vi "cs-scanning-dirty.vi"() -> ()   [LabVIEW 2017]
uses:
  raster-scan-params.ctl
  controls/PI-params.ctl
  controls/boolean_info.ctl
  <vilib>/rvi/Emulation/niFpgaGetClockAttributes.vi
  <vilib>/rvi/Emulation/niFpgaSctlEmulationGetInTimedLoop.vi
  <vilib>/rvi/Emulation/niFpgaEmulationReportErrorSimple.vi
  <vilib>/rvi/Emulation/niFpgaProcessEmulError.vi
  <vilib>/rvi/eio/common/nirviEmuTemplateMethod_errors.vi
  <vilib>/rvi/Emulation/niFpgaEmulationIsFPGAContextNoSignature.vi
  <vilib>/rvi/DataTransferAndStorage/Container/Common/niFpgaContainerGetUniqueNameForEmu.vi
  <vilib>/rvi/Memory/Memory_Emulation/niFpgaMemoryEmulationCacheClearOnFirstRun.vi
  <vilib>/rvi/Memory/Memory_Emulation/nirvimemoryEmulationManagerCache_MakeExclusive.vi
  <vilib>/rvi/Memory/Memory_Emulation/niFpgaMemoryEmulationValidateCache.vi
  <vilib>/rvi/Memory/Memory_Emulation/nirvimemoryEmulationManagerCache_InsertValue.vi
  <vilib>/Utility/error.llb/Clear Errors.vi
  <vilib>/rvi/Memory/Memory_Emulation/nirvimemoryEmulationManagerCache_ReleaseExclusive.vi
  <vilib>/rvi/Memory/Memory_Emulation/nirvimemoryEmulationManagerCache_GetValue.vi
  <vilib>/rvi/Memory/Memory_Emulation/nirvimemoryEmulationManagerCache_SetValue.vi
  <vilib>/rvi/DataTransferAndStorage/Container/Common/niFpgaContainerExecOnDevCompGetState.vi
  <vilib>/rvi/Emulation/niFpgaCriticalErrorInLSC.vi
  <vilib>/eio/EIONode/EIONode.xnode
  <vilib>/rvi/DataTransferAndStorage/Container/XNode/niFpgaContainer.xnode
  <vilib>/rvi/DataTransferAndStorage/Register/Emulation/niFpgaRegisterEmulation.vi
  <vilib>/rvi/DataTransferAndStorage/Register/Emulation/niFpgaRegisterEmulationRefIn.vi
  libimaging-cs.lvlib
  FPGA-data-logging.lvlib
panel:
  out "number-settled-samples-Z":i16
  in  "Z-error-threshold":sgl format="%#_13g"
  in  "Z-settled-samples\nthreshold":i16
  out "number-settled-samples-y":i16
  out "number-settled-samples-x":i16
  in  "error-threshold":sgl format="%#_13g"
  in  "settled-samples\nthreshold":i16
  out "case-selected":i16
  out "z-DAC":sgl
  in  "numEntities":i16
  in  "ABORT":bool
  in  "Ki-xy":sgl=0.001 format="%#_13g"
  in  "z-bound":sgl
  in  "xy-bound":sgl
  out "boolean indicators":T1
  out "loggin-fifo-TO":bool=TRUE
  out "input-fifo-TO":bool=TRUE
  in  "raster-scan-params":T2={"TsTicks"=1600, "Stop"=TRUE, "TOL"=0.3, "ramp-rate"=0.0, "z-u-max"=5.0, "PI-params"={"Ki"=0.001, "setpoint"=0.0}} {"z-u-max" format="%#_13g"; "TOL" format="%#_13g"}
  in  "init Z up":fxp<+/-,16,5>
  in  "u_z(0)":sgl
  out "ADC-zaxis":fxp<+/-,24,5>
  out "e(0) (threshhold init)":fxp<+/-,16,5>
  out "xref ?":sgl=0.001 format="%#_13g"
  in  "z_UP":fxp<+/-,16,5>
  in  "zup-N":i16
  out "yref ?":sgl=0.001 format="%#_13g"
  in  "trigger-0":bool
  in  "initial case":i16=2
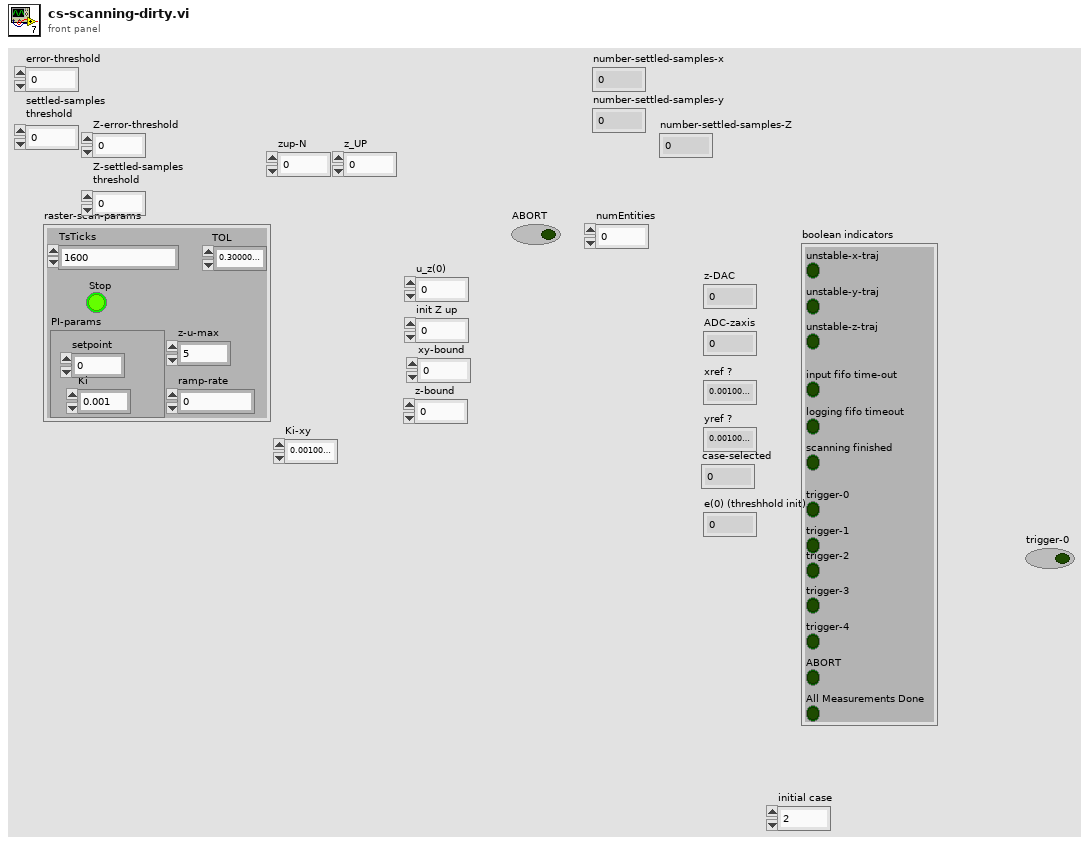
[diagram p1: front panel]
types:
  T1 = typedef "boolean_info.ctl" = cluster{"unstable-z-traj":bool, "input fifo time-out":bool, "logging fifo timeout":bool, "scanning finished":bool, "trigger-1":bool, "trigger-0":bool, "trigger-2":bool, "trigger-3":bool, "trigger-4":bool, "unstable-x-traj":bool, "unstable-y-traj":bool, "ABORT":bool, "All Measurements Done":bool}
  T2 = typedef "raster-scan-params.ctl" = cluster{"TsTicks":u32, "Stop":bool, "TOL":sgl, "ramp-rate":sgl, "z-u-max":sgl, "PI-params":T3}
  T3 = typedef "PI-params.ctl" = cluster{"Ki":sgl, "setpoint":sgl}
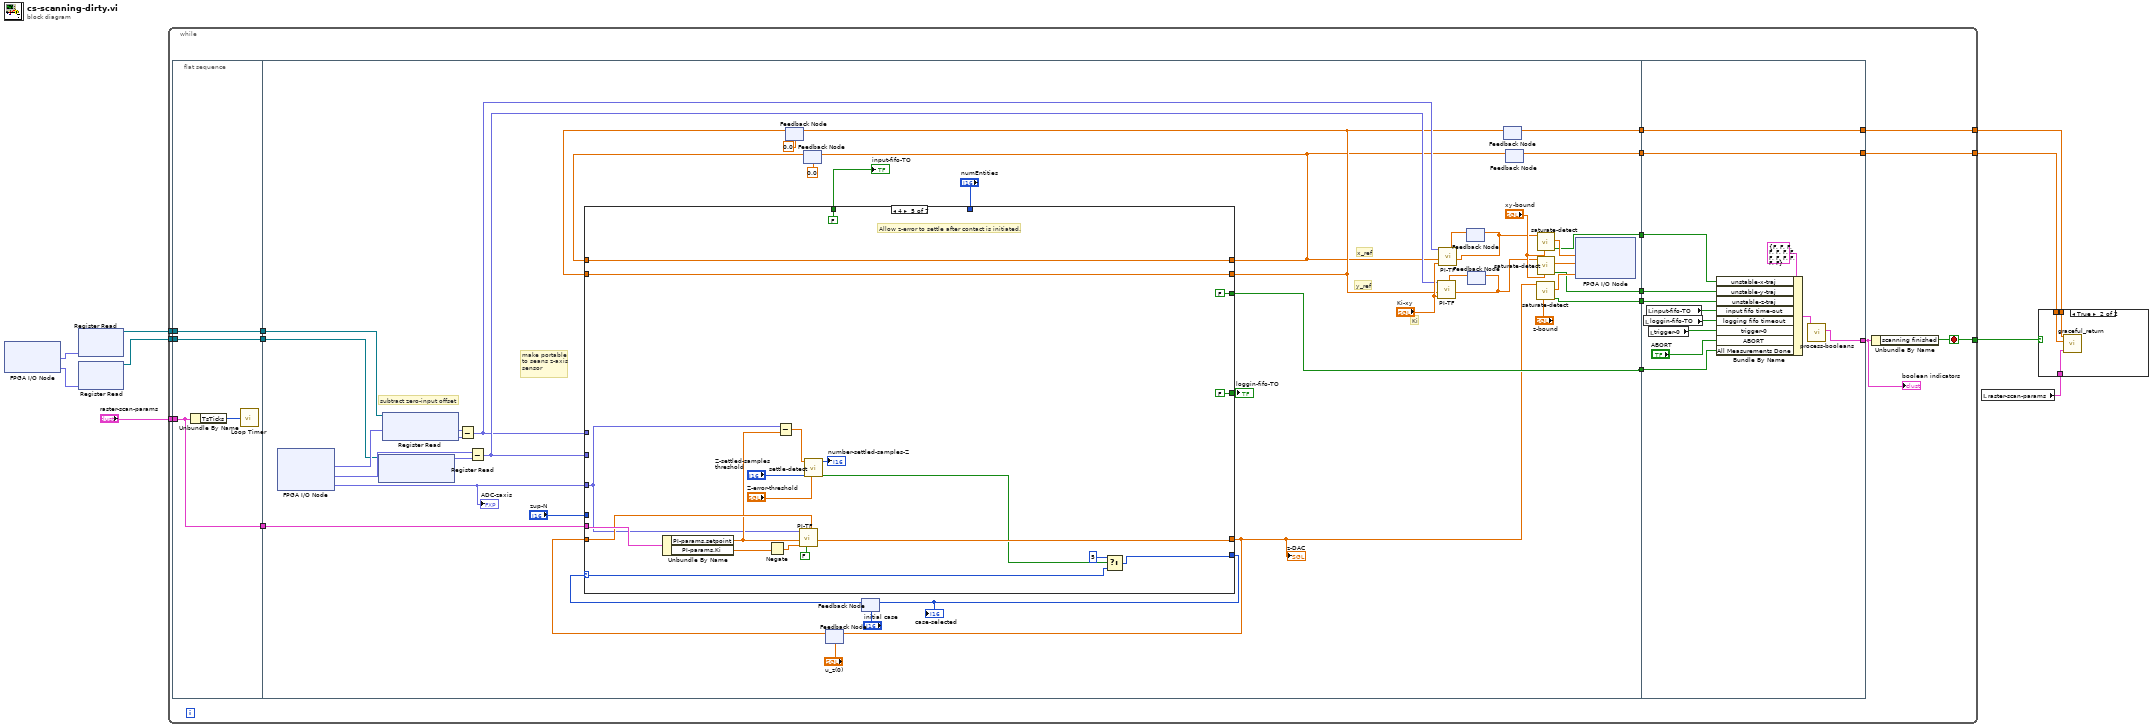
[diagram p0: block diagram]
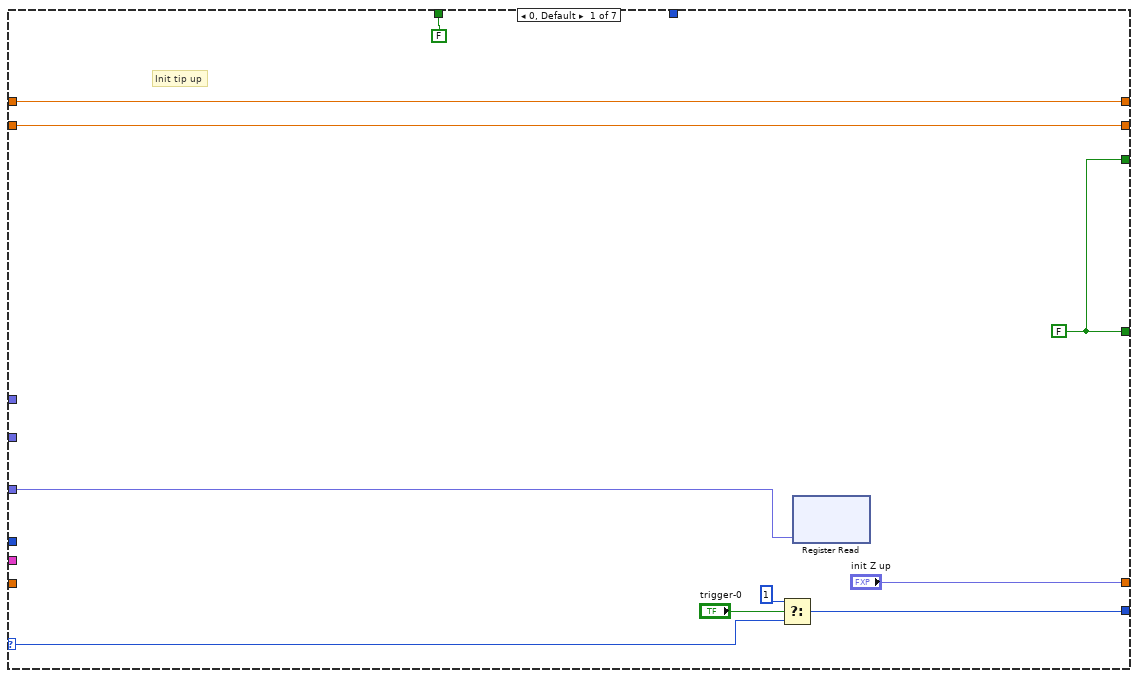
[diagram p3: hidden frame]
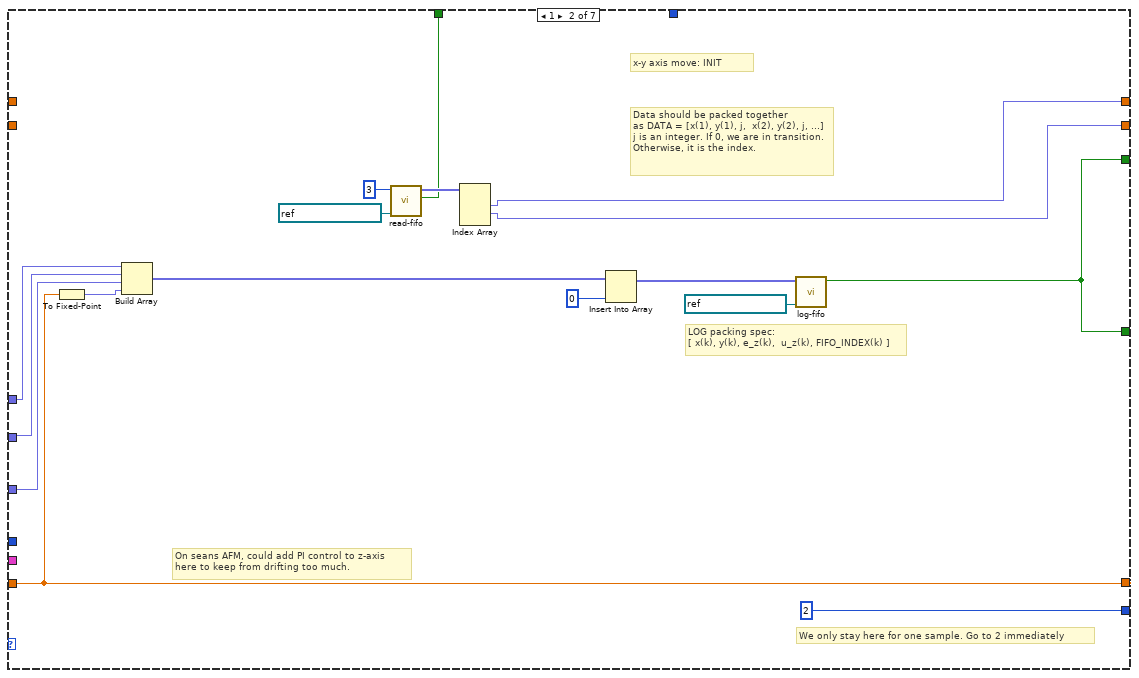
[diagram p4: hidden frame]
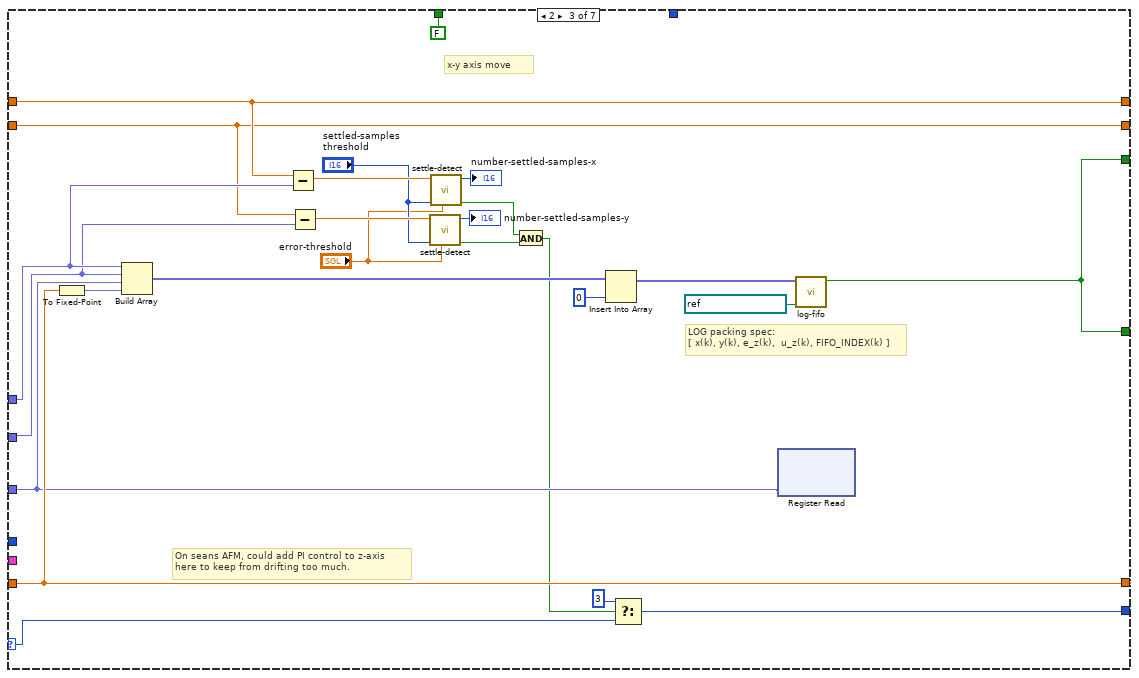
[diagram p5: hidden frame]
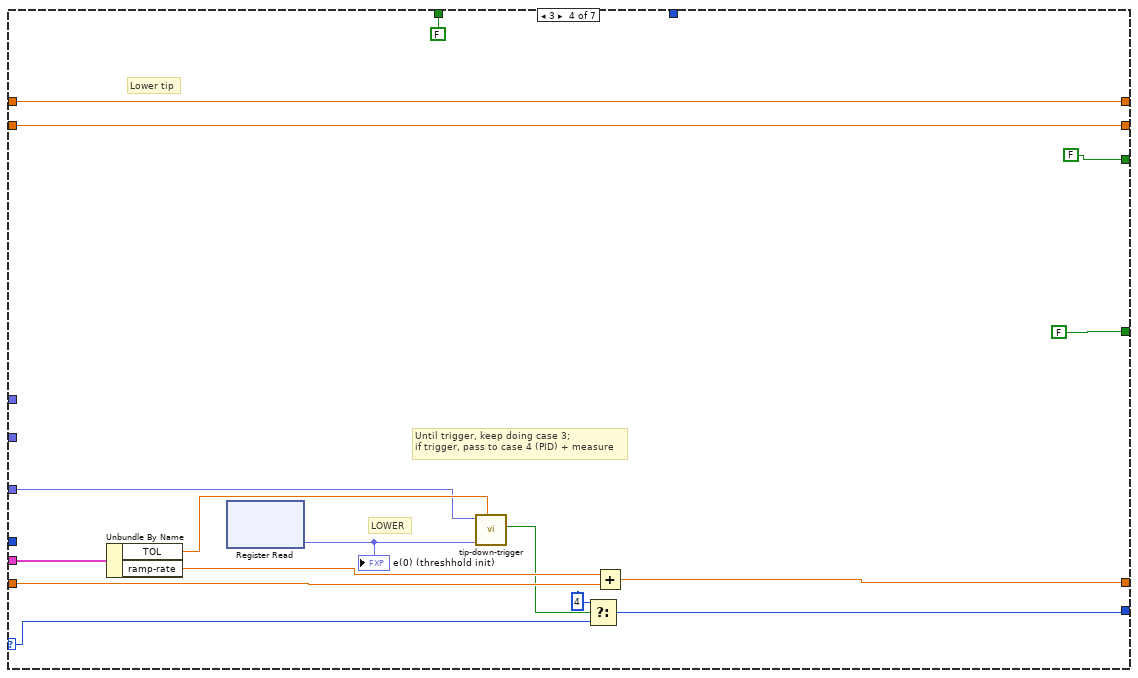
[diagram p6: hidden frame]
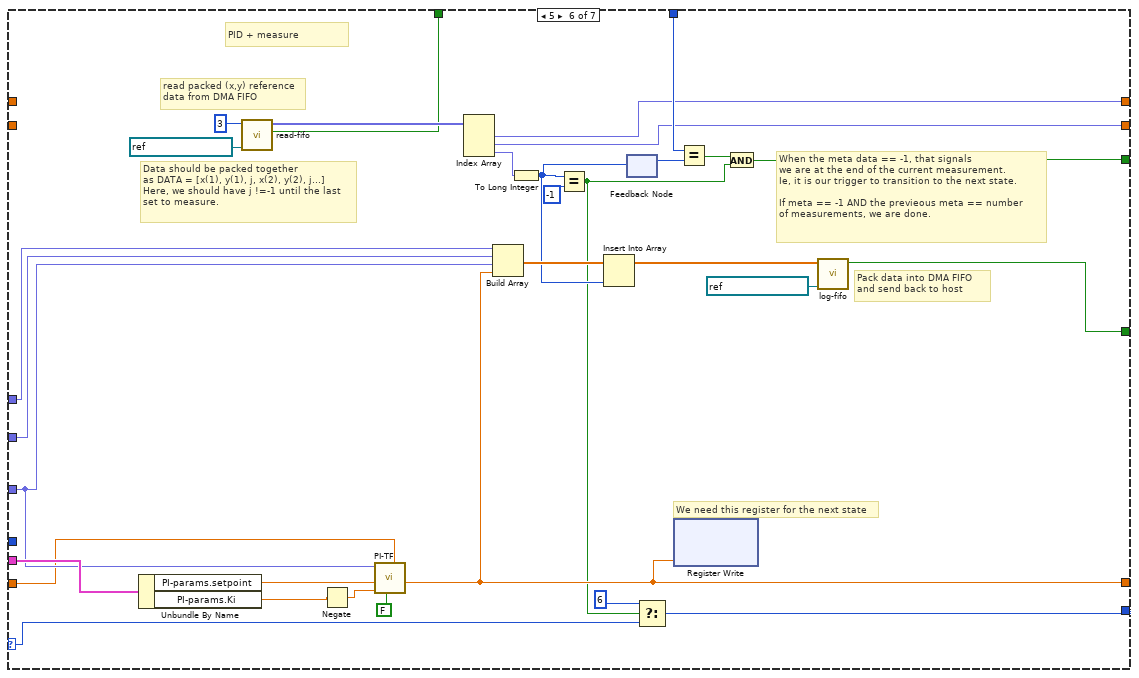
[diagram p7: hidden frame]
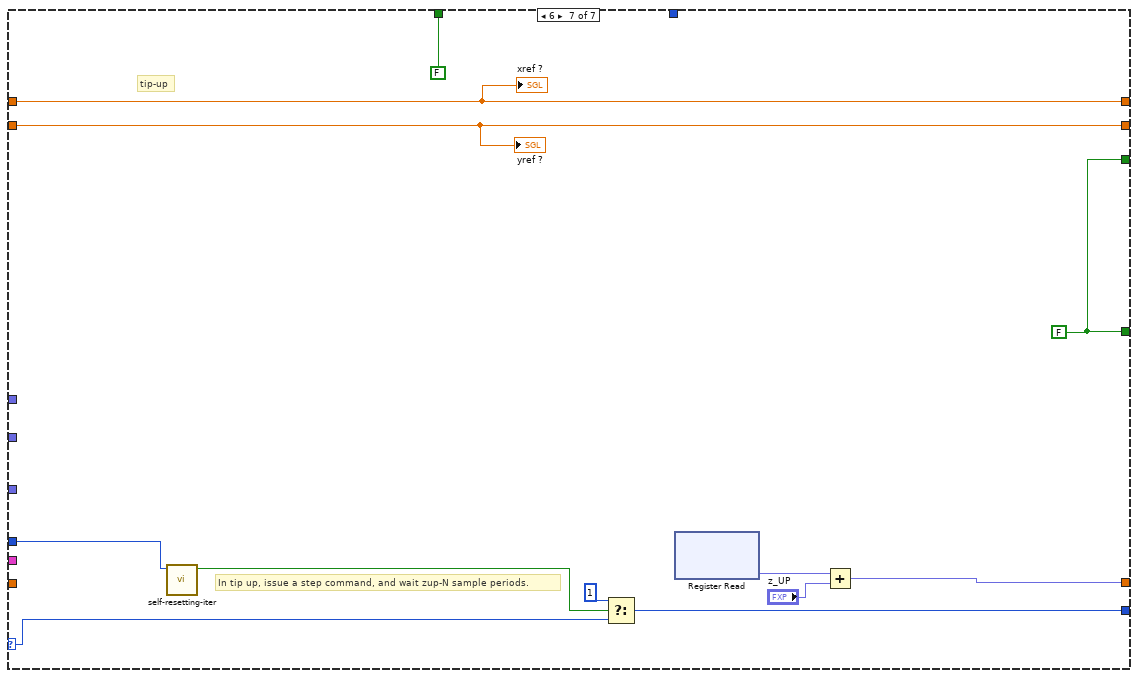
[diagram p8: hidden frame]
diagram:
  n1 = xnode "FPGA I/O Node"() -> ("Mod2/AI0"=w4:fxp<+/-,24,5>, "Mod2/AI1"=w3:fxp<+/-,24,5>)  [unwired: 2 in, 2 out]
  n2 = xnode ("Register Read")("Data"=w3) -> ("Register Out"=w1:refnum<k21>)  [unwired: 1 in]
  n3 = xnode ("Register Read")("Data"=w4) -> ("Register Out"=w2:refnum<k21>)  [unwired: 1 in]
  n4 = while {
    tunnel: "raster-scan-params" -> [w24]
    tunnel: [w23] -> w6
    tunnel: [w22] -> w7
    tunnel: [w19] -> w5
    tunnel: w2 -> [w12]
    tunnel: w1 -> [w10]
    stop <- w19 stop-if-true
    n5 = flat-sequence {
      tunnel: w24 -> [w28]
      tunnel: [w28] -> w25
      tunnel: [w27] -> w13
      tunnel: w12 -> [w27]
      tunnel: [w26] -> w11
      tunnel: w10 -> [w26]
      tunnel: w25 -> [w55]
      tunnel: [w52] -> w21
      tunnel: [w51] -> w20
      tunnel: [w43] -> w17
      tunnel: [w42] -> w16
      tunnel: [w41] -> w15
      tunnel: [w37] -> w14
      tunnel: w13 -> [w36]
      tunnel: w11 -> [w35]
      tunnel: [w215] -> w22
      tunnel: [w216] -> w23
      tunnel: w21 -> [w216]
      tunnel: w20 -> [w215]
      tunnel: [w207] -> w18
      tunnel: w17 -> [w211]
      tunnel: w16 -> [w210]
      tunnel: w15 -> [w209]
      tunnel: w14 -> [w206]
      frame #0 {
        n6 = Unbundle By Name(w28) -> ("TsTicks"=w29:u32)
        n7 = call "Loop Timer"("Count(Ticks)"=w29) -> ()  [unwired: 1 out]
      }
      frame #1 {
        # "make portable\nto seans z-axis\nsensor"
        # "subtract zero-input offset"
        # "x_ref"
        # "y_ref"
        # "Ki"
        n8 = xnode "FPGA I/O Node"() -> ("Mod2/AI0"=w61:fxp<+/-,24,5>, "Mod2/AI1"=w59:fxp<+/-,24,5>, "Mod2/AI2"=w30:fxp<+/-,24,5>)  [unwired: 3 in, 3 out]
        "ADC-zaxis" <- w30
        n9 = xnode ("Register Read")("Register In"=w35) -> ("Data"=w58:fxp<+/-,16,5>)  [unwired: 1 out]
        n10 = xnode ("Register Read")("Register In"=w36) -> ("Data"=w60:fxp<+/-,16,5>)  [unwired: 1 out]
        n11 = Subtract(x=w61, y=w60) -> (x-y=w56:fxp<+/-,25,6>)
        n12 = Subtract(x=w59, y=w58) -> (x-y=w57:fxp<+/-,25,6>)
        n13 = feedback #1(sgl 0.0) -> (w64:sgl)
        n14 = feedback #2(sgl 0.0) -> (w63:sgl)
        n15 = feedback #3("u_z(0)") -> (w33:sgl)
        n16 = feedback #4("initial case") -> (w70:i16)
        n17 = case shown="4" w70 {
          selector: w70 -> [w72 _ w99 w126 w149 w171 w192]
          tunnel: [w80 i16 2 w123 w138 w147 w190 w202] -> w31
          tunnel: w57 -> [_ w96 w107 _ _ w178 _]
          tunnel: w30 -> [w76 w94 w119 w124 w143 w177 _]
          tunnel: ["init Z up" w98 w121 w130 w155 w169 w198] -> w32
          tunnel: [w79 w83 w103 w137 w142 w162 w200] -> w53
          tunnel: [w78 w82 w102 w136 w141 w161 w199] -> w54
          tunnel: w64 -> [w78 _ w102 w136 w141 _ w199]
          tunnel: w63 -> [w79 _ w103 w137 w142 _ w200]
          tunnel: w55 -> [_ _ _ w133 w157 w185 _]
          tunnel: w33 -> [_ w98 w121 w132 w156 w176 _]
          tunnel: w56 -> [_ w95 w109 _ _ w179 _]
          tunnel: [w74 w86 w115 FALSE FALSE ("logging-timeout?") w180 w195] -> w40
          tunnel: [FALSE w89 FALSE ("timout?") FALSE FALSE ("timout?") w182 FALSE] -> w39
          tunnel: "numEntities" -> [_ _ _ _ _ w168 _]
          tunnel: [w74 w86 w115 FALSE FALSE ("logging-timeout?") w163 w195] -> w37
          tunnel: "zup-N" -> [_ _ _ _ _ _ w194]
          frame 0, Default {
            w74 = FALSE
            # "Init tip up"
            n18 = Select(t=i16 1, s="trigger-0", f=w72) -> (s? t:f=w80:i16)
            n19 = xnode ("Register Read")("Data"=w76) -> ()  [unwired: 1 in, 1 out]
          }
          frame 1 {
            # "We only stay here for one sample. Go to 2 immediately"
            # "LOG packing spec:\n[ x(k), y(k), e_z(k),  u_z(k), FIFO_INDEX(k) ]"
            # "On seans AFM, could add PI control to z-axis\nhere to keep from drifting too much."
            # "Data should be packed together\nas DATA = [x(1), y(1), j,  x(2), y(2), j, ...]\nj is an integer. If 0, we are in transition. Otherwise, it is the index."
            # "x-y axis move: INIT"
            n20 = To Fixed-Point(number=w98) -> (fixed-point=w93:fxp<+/-,16,5>)  [unwired: 1 in]
            n21 = Build Array(w95, w96, w94, w93) -> (w97:fxp<+/-,25,6>[])
            n22 = call "read-fifo.vi"("FIFO In"=refnum<k21> "Host_to_FPGA", "numChan"=3) -> ("timout?"=w89:bool, "unpacked-data"=w90:fxp<+/-,16,5>[])  [unwired: 8 in]
            n23 = Index Array(array=w90) -> (element #1=w83:fxp<+/-,16,5>, element #2=w82:fxp<+/-,16,5>)  [unwired: 3 in, 1 out]
            n24 = Insert Into Array(array=w97, new element=0 ("numChan")) -> (w88:fxp<+/-,25,6>[])  [unwired: 1 in]
            n25 = call "log-fifo.vi"("FIFO In"=refnum<k21> "fpga-to-host2", "input-data"=w88) -> ("logging-timeout?"=w86:bool)  [unwired: 9 in]
          }
          frame 2 {
            # "LOG packing spec:\n[ x(k), y(k), e_z(k),  u_z(k), FIFO_INDEX(k) ]"
            # "On seans AFM, could add PI control to z-axis\nhere to keep from drifting too much."
            # "x-y axis move"
            n26 = To Fixed-Point(number=w121) -> (fixed-point=w118:fxp<+/-,16,5>)  [unwired: 1 in]
            n27 = Build Array(w109, w107, w119, w118) -> (w120:fxp<+/-,25,6>[])
            n28 = Subtract(x=w103, y=w109) -> (x-y=w110:sgl)
            n29 = Subtract(x=w102, y=w107) -> (x-y=w108:sgl)
            n30 = call "settle-detect.vi"("error-max"="error-threshold", "settled-samples\nthreshold"="settled-samples\nthreshold", "err(k)"=w108) -> ("has-settled"=w112:bool, "number-settled-samples"=→"number-settled-samples-y":i16)  [unwired: 7 in]
            n31 = call "settle-detect.vi"("error-max"="error-threshold", "settled-samples\nthreshold"="settled-samples\nthreshold", "err(k)"=w110) -> ("has-settled"=w111:bool, "number-settled-samples"=→"number-settled-samples-x":i16)  [unwired: 7 in]
            n32 = And(x=w111, y=w112) -> (x .and. y?=w104:bool)
            n33 = Insert Into Array(array=w120, new element=i16 0) -> (w117:fxp<+/-,25,6>[])  [unwired: 1 in]
            n34 = Select(t=i16 3, s=w104, f=w99) -> (s? t:f=w123:i16)
            n35 = xnode ("Register Read")("Data"=w119) -> ()  [unwired: 1 in, 1 out]
            n36 = call "log-fifo.vi"("FIFO In"=refnum<k21> "fpga-to-host2", "input-data"=w117) -> ("logging-timeout?"=w115:bool)  [unwired: 9 in]
          }
          frame 3 {
            # "Until trigger, keep doing case 3;\nif trigger, pass to case 4 (PID) + measure"
            # "LOWER"
            # "Lower tip"
            n37 = Unbundle By Name(w133) -> ("TOL"=w134:sgl, "ramp-rate"=w127:sgl)
            n38 = xnode ("Register Read")() -> ("Data"=w135:fxp<+/-,16,5>)  [unwired: 1 in, 1 out]
            "e(0) (threshhold init)" <- w135
            n39 = call "tip-down-trigger.vi"("TOL"=w134, "Vo"=w135, "e(k)"=w124) -> ("trigger"=w125:bool)  [unwired: 8 in]
            n40 = Select(t=i16 4, s=w125, f=w126) -> (s? t:f=w138:i16)
            n41 = Add(x=w127, y=w132) -> (x+y=w130:sgl)
          }
          frame 4 {
            # "Allow z-error to settle after contact is initiated."
            n42 = Unbundle By Name(w157) -> ("PI-params.setpoint"=w151:sgl, "PI-params.Ki"=w158:sgl)
            n43 = Negate(x=w158) -> (-x=w159:sgl)
            n44 = Subtract(x=w143, y=w151) -> (x-y=w152:sgl)
            n45 = call "PI-TF.vi"("u(k-1)"=w156, "reset"=FALSE, "Ki"=w159, "setpoint"=w151, "y(k)"=w143) -> ("u(k)"=w155:sgl)  [unwired: 6 in]
            n46 = call "settle-detect.vi"("error-max"="Z-error-threshold", "settled-samples\nthreshold"="Z-settled-samples\nthreshold", "err(k)"=w152) -> ("has-settled"=w148:bool, "number-settled-samples"=→"number-settled-samples-Z":i16)  [unwired: 7 in]
            n47 = Select(t=i16 5, s=w148, f=w149) -> (s? t:f=w147:i16)
          }
          frame 5 {
            # "Pack data into DMA FIFO\nand send back to host"
            # "read packed (x,y) reference\ndata from DMA FIFO"
            # "When the meta data == -1, that signals\nwe are at the end of the current measurement.\nIe, it is our trigger to transition to the next state.\n\nIf meta == -1 AND the previeous meta == number\nof measurements, we are done."
            # "We need this register for the next state"
            # "Data should be packed together\nas DATA = [x(1), y(1), j, x(2), y(2), j...]\nHere, we should have j !=-1 until the last\nset to measure."
            # "PID + measure"
            n48 = Unbundle By Name(w185) -> ("PI-params.setpoint"=w186:sgl, "PI-params.Ki"=w183:sgl)
            n49 = call "read-fifo.vi"("FIFO In"=refnum<k21> "Host_to_FPGA", "numChan"=3) -> ("timout?"=w182:bool, "unpacked-data"=w189:fxp<+/-,16,5>[])  [unwired: 8 in]
            n50 = Negate(x=w183) -> (-x=w184:sgl)
            n51 = call "PI-TF.vi"("u(k-1)"=w176, "reset"=FALSE, "Ki"=w184, "setpoint"=w186, "y(k)"=w177) -> ("u(k)"=w169:sgl)  [unwired: 6 in]
            n52 = Index Array(array=w189) -> (element #1=w162:fxp<+/-,16,5>, element #2=w161:fxp<+/-,16,5>, element #3=w188:fxp<+/-,16,5>)  [unwired: 3 in]
            n53 = Build Array(w179, w178, w177, w169) -> (w175:sgl[])
            n54 = To Long Integer(number=w188) -> (32bit integer=w166:i32)
            n55 = Equal?(x=w166, y=-1) -> (x = y?=w164:bool)
            n56 = Insert Into Array(array=w175, new element=w166) -> (w181:sgl[])  [unwired: 1 in]
            n57 = feedback-in #5(w166) -> ()
            n58 = feedback #5() -> (w167:i32)  [unwired: 1 in]
            n59 = Select(t=i16 6, s=w164, f=w171) -> (s? t:f=w190:i16)
            n60 = xnode ("Register Write")("Data"=w169) -> ()  [unwired: 1 in, 1 out]
            n61 = Equal?(x=w168, y=w167) -> (x = y?=w165:bool)
            n62 = And(x=w165, y=w164) -> (x .and. y?=w163:bool)
            n63 = call "log-fifo.vi"("FIFO In"=refnum<k21> "fpga-to-host2", "input-data"=w181) -> ("logging-timeout?"=w180:bool)  [unwired: 9 in]
          }
          frame 6 {
            w195 = FALSE
            # "In tip up, issue a step command, and wait zup-N sample periods."
            # "tip-up"
            n64 = call "self-resetting-iter.vi"("N"=w194) -> ("Boolean"=w193:bool)  [unwired: 9 in, 1 out]
            n65 = Select(t=i16 1, s=w193, f=w192) -> (s? t:f=w202:i16)
            n66 = xnode ("Register Read")() -> ("Data"=w196:fxp<+/-,16,5>)  [unwired: 1 in, 1 out]
            n67 = Add(x=w196, y="z_UP") -> (x+y=w198:fxp<+/-,17,6>)
            "yref ?" <- w199
            "xref ?" <- w200
          }
        }
        "loggin-fifo-TO" <- w40
        "input-fifo-TO" <- w39
        "z-DAC" <- w32
        "case-selected" <- w31
        n68 = feedback-in #1(w54) -> ()
        n69 = feedback-in #2(w53) -> ()
        n70 = feedback-in #3(w32) -> ()
        n71 = feedback-in #4(w31) -> ()
        n72 = feedback #6() -> (w68:sgl)  [unwired: 1 in]
        n73 = call "PI-TF.vi"("u(k-1)"=w68, "Ki"="Ki-xy", "setpoint"=w53, "y(k)"=w56) -> ("u(k)"=w46:sgl)  [unwired: 7 in]
        n74 = feedback-in #6(w46) -> ()
        n75 = feedback #7() -> (w67:sgl)  [unwired: 1 in]
        n76 = call "PI-TF.vi"("u(k-1)"=w67, "Ki"="Ki-xy", "setpoint"=w54, "y(k)"=w57) -> ("u(k)"=w47:sgl)  [unwired: 7 in]
        n77 = feedback-in #7(w47) -> ()
        n78 = feedback #8() -> (w51:sgl)  [unwired: 1 in]
        n79 = feedback-in #8(w54) -> ()
        n80 = feedback #9() -> (w52:sgl)  [unwired: 1 in]
        n81 = feedback-in #9(w53) -> ()
        n82 = call "saturate-detect.vi"("bound"="z-bound", "x"=w32) -> ("saturated"=w41:bool, "sat(x)"=w45:sgl)  [unwired: 8 in]
        n83 = call "saturate-detect.vi"("bound"="xy-bound", "x"=w46) -> ("saturated"=w43:bool, "sat(x)"=w48:sgl)  [unwired: 8 in]
        n84 = call "saturate-detect.vi"("bound"="xy-bound", "x"=w47) -> ("saturated"=w42:bool, "sat(x)"=w49:sgl)  [unwired: 8 in]
        n85 = xnode "FPGA I/O Node"("Mod1/AO0"=w48, "Mod1/AO1"=w49, "Mod1/AO2"=w45) -> ()  [unwired: 3 in, 3 out]
      }
      frame #2 {
        n86 = local read "loggin-fifo-TO"() -> (w213:bool)
        n87 = local read "input-fifo-TO"() -> (w214:bool)
        n88 = local read "trigger-0"() -> (w212:bool)
        n89 = Bundle By Name(cluster=T1 {"unstable-z-traj"=FALSE, "input fifo time-out"=FALSE, "logging fifo timeout"=FALSE, "scanning finished"=FALSE, "trigger-1"=FALSE, "trigger-0"=FALSE, "trigger-2"=FALSE, "trigger-3"=FALSE, "trigger-4"=FALSE, "unstable-x-traj"=FALSE, "unstable-y-traj"=FALSE, "ABORT"=FALSE, "All Measurements Done"=FALSE} ("boolean errors"), "unstable-x-traj"=w211, "unstable-y-traj"=w210, "unstable-z-traj"=w209, "input fifo time-out"=w214, "logging fifo timeout"=w213, "trigger-0"=w212, "ABORT"="ABORT", "All Measurements Done"=w206) -> (w205:T1)
        n90 = call "process-booleans.vi"("boolean indicators 2"=w205) -> ("boolean indicators"=w207:T1)  [unwired: 9 in, 1 out]
      }
    }
    n91 = Unbundle By Name(w18) -> ("scanning finished"=w19:bool)
    "boolean indicators" <- w18
  }
  n92 = local read "raster-scan-params"() -> (w8:T2)
  n93 = case shown="True" w5 {
    tunnel: w7 -> [_ w219]
    tunnel: w6 -> [_ w218]
    tunnel: w8 -> [_ w217]
    frame False {
    }
    frame True {
      n94 = call "graceful_return.vi"("raster-scan-params"=w217, "uy(0)"=w218, "ux(0)"=w219) -> ()  [unwired: 9 in]
    }
  }
